vi "Reset Output Protection Core.vi"(8 "error in (no error)":errorcluster, 10 "channel name (\"CHANNEL1\")":string="CHANNEL1", 11 "CS++DCPwr in":refnum<class "CS++DCPwr.lvclass">) -> (0 "error out":errorcluster, 3 "CS++DCPwr out":refnum<class "CS++DCPwr.lvclass">)   [LabVIEW 2016, in "CS++DCPwr.lvlib" / "CS++DCPwr.lvclass"]
doc: "This VI clears all output-protection conditions on the power supply."
uses:
  CS++DCPwr.lvclass
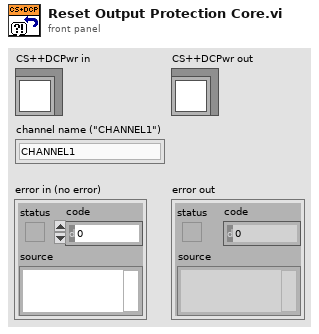
[diagram p1: front panel]
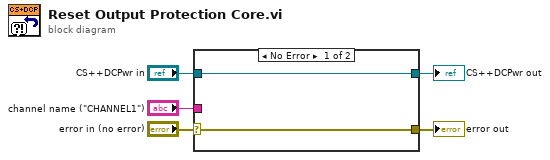
[diagram p0: block diagram]
diagram:
  n1 = case shown="No Error" "error in (no error)" {
    selector: "error in (no error)" -> [w6 w9]
    tunnel: [w6 w9] -> w4
    tunnel: [w7 w8] -> w2
    tunnel: "CS++DCPwr in" -> [w7 w8]
    tunnel: "channel name (\"CHANNEL1\")" -> [_ _]
    frame No Error {
    }
    frame Error {
    }
  }
  "error out" <- w4
  "CS++DCPwr out" <- w2
